vi "writeANDupdate_rownumber.vi"(8 "error in (no error)":errorcluster, 11 "reference":refnum<vi>) -> (0 "error out":errorcluster, 3 "reference out":refnum<vi>)   [LabVIEW 2022 SP3]
uses:
  <vilib>/Utility/miscctls.llb/LVRowAndColumnUnsignedTypeDef.ctl
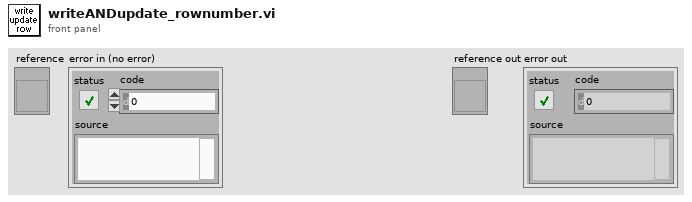
[diagram p1: front panel]
types:
  T1 = typedef "LVRowAndColumnUnsignedTypeDef.ctl" = cluster{"Row":u32, "Column":u32}
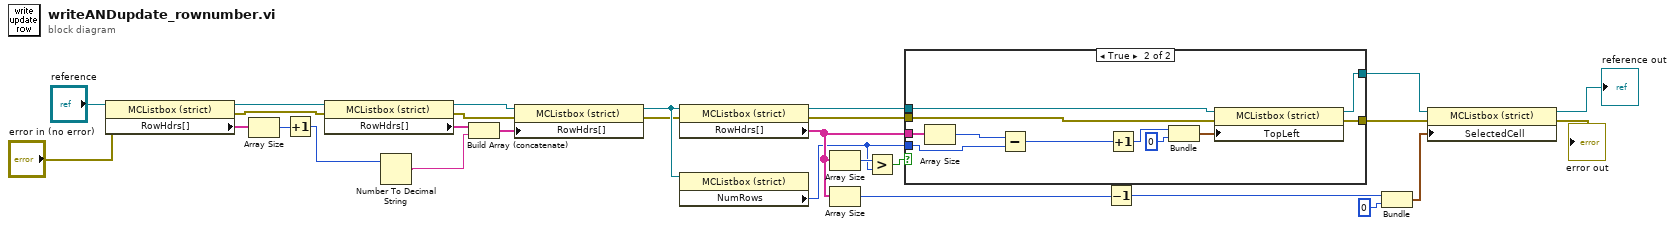
[diagram p0: block diagram]
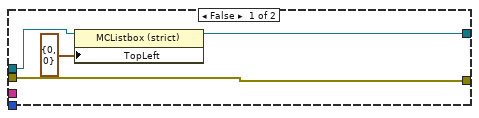
[diagram p2: hidden frame]
diagram:
  n1 = property on="Property Node" class="MCListbox (strict)"(reference="reference", error in="error in (no error)") -> (reference out=w21:refnum<vi>, error out=w19:errorcluster, "RowHdrs[]"=w25:string[])
  n2 = Array Size(array=w25) -> (size(s)=w22:i32)
  n3 = Increment(x=w22) -> (x+1=w28:i32)
  n4 = property on="Property Node" class="MCListbox (strict)"(reference=w21, error in=w19) -> (reference out=w20:refnum<vi>, error out=w18:errorcluster, "RowHdrs[]"=w24:string[])
  n5 = Number To Decimal String(number=w28) -> (decimal integer string=w27:string)  [unwired: 1 in]
  n6 = Build Array (concatenate)(w24, w27) -> (w23:string[])
  n7 = property on="Property Node" class="MCListbox (strict)"(reference=w20, error in=w18, "RowHdrs[]"=w23) -> (reference out=w26:refnum<vi>, error out=w1:errorcluster)
  n8 = property class="MCListbox (strict)"(reference=w26, error in=w1) -> (reference out=w6:refnum<vi>, error out=w7:errorcluster, "RowHdrs[]"=w12:string[])
  n9 = property class="MCListbox (strict)"(reference=w26) -> ("NumRows"=w8:u32)  [unwired: 1 in, 2 out]
  n10 = Array Size(array=w12) -> (size(s)=w9:i32)
  n11 = Array Size(array=w12) -> (size(s)=w13:i32)
  n12 = Greater?(x=w9, y=w8) -> (0:w10:bool)
  n13 = case shown="True" w10 {
    tunnel: w6 -> [w30 w43]
    tunnel: w7 -> [w32 w42]
    tunnel: w12 -> [_ w39]
    tunnel: w8 -> [_ w36]
    tunnel: [w29 w38] -> w16
    tunnel: [w32 w35] -> w11
    frame False {
      n14 = property class="MCListbox (strict)"(reference=w30, "TopLeft"=T1 {"Row"=0, "Column"=0} ("Top Left Visible Cell")) -> (reference out=w29:refnum<vi>)  [unwired: 1 in, 1 out]
    }
    frame True {
      n15 = Array Size(array=w39) -> (size(s)=w37:i32)
      n16 = Subtract(x=w37, y=w36) -> (x-y=w34:u32)
      n17 = Increment(x=w34) -> (x+1=w33:u32)
      n18 = Bundle(w33, "Number of Rows"=u32 0) -> (w41:cluster{u32, "Number of Rows":u32})  [unwired: 1 in]
      n19 = property class="MCListbox (strict)"(reference=w43, error in=w42, "TopLeft"=w41) -> (reference out=w38:refnum<vi>, error out=w35:errorcluster)
    }
  }
  n20 = Decrement(x=w13) -> (x-1=w17:i32)
  n21 = Bundle(w17, "Number of Rows"=u32 0) -> (w15:cluster{i32, "Number of Rows":u32})  [unwired: 1 in]
  n22 = property class="MCListbox (strict)"(reference=w16, error in=w11, "SelectedCell"=w15) -> (reference out=→"reference out":refnum<vi>, error out=→"error out":errorcluster)
